vi "Enqueue.vi"(4 "Frist Call (F)":bool, 5 "QueueNames In":string[](array[string]), 6 "EnqueueType (QMH)":T2, 7 "EnqueueType (Enqueue)":T1=enum."Enqueue", 8 "error in (no error)":errorcluster, 9 "Message Data":variant, 10 "Message":string, 11 "Queue Array Reference In":refnum<queue>[](array[refnum])) -> (0 "error out":errorcluster, 2 "Queue Array Reference Out":refnum<queue>[](array[refnum]), 3 "MessageQueue":refnum<queue>)   [LabVIEW 2018, in "ScopePlugins.lvlib"]
uses:
  ScopePlugins.lvlib
  clMessage.ctl
  TypeDefs/QueueNames.ctl
  EnqueueTypes.ctl
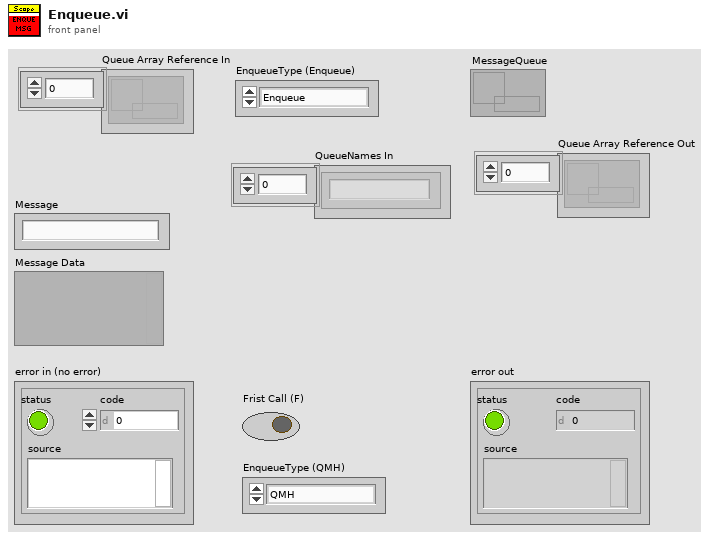
[diagram p1: front panel]
types:
  T1 = typedef "ScopePlugins.lvlib/EnqueueTypes.ctl" = enum16{"LossyEnqueue", "EnqueueAtFront", "Enqueue"}
  T2 = typedef "ScopePlugins.lvlib/QueueNames.ctl" = enum16{"QMH", "Class ", "MA"}
  T3 = typedef "ScopePlugins.lvlib/clMessage.ctl" = cluster{"Message":string, "Message Data":variant}
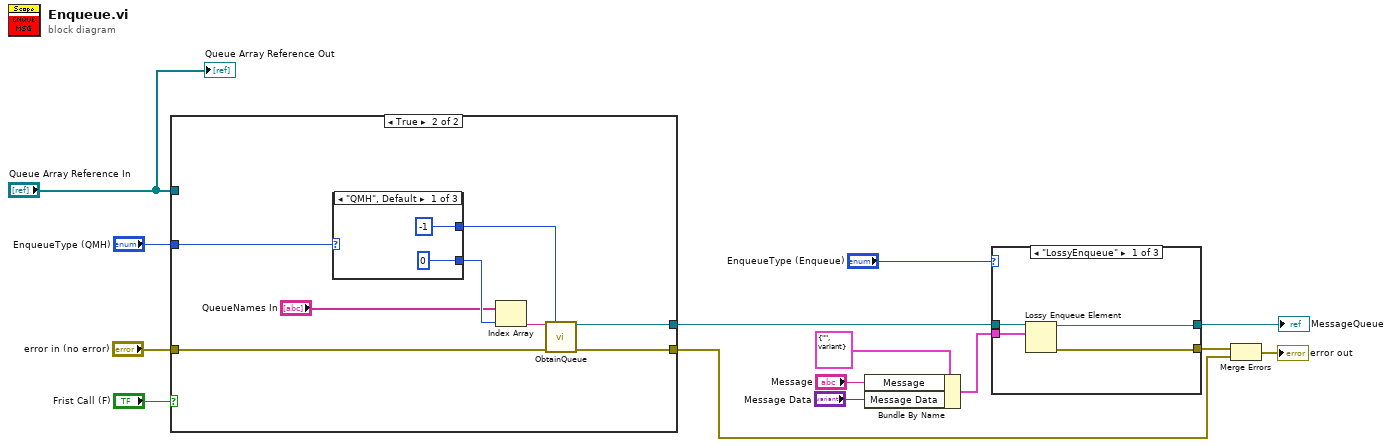
[diagram p0: block diagram]
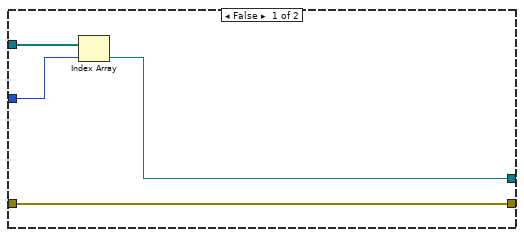
[diagram p2: hidden frame]
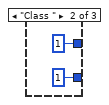
[diagram p3: hidden frame]
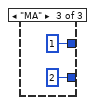
[diagram p4: hidden frame]
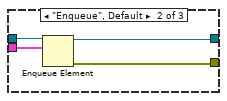
[diagram p5: hidden frame]
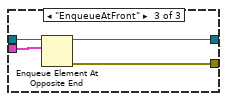
[diagram p6: hidden frame]
diagram:
  n1 = case shown="True" "Frist Call (F)" {
    tunnel: [w17 w26] -> w7
    tunnel: [w16 w25] -> w6
    tunnel: "EnqueueType (QMH)" -> [w18 w20]
    tunnel: "error in (no error)" -> [w16 w19]
    tunnel: "Queue Array Reference In" -> [w15 _]
    frame False {
      n2 = Index Array(array=w15, index=w18) -> (element=w17:refnum<queue>)
    }
    frame True {
      n3 = case shown="\"QMH\", Default" w20 {
        tunnel: [-1 ("max queue size (-1, unlimited)") 1 ("max queue size (-1, unlimited)") 1 ("max queue size (-1, unlimited)")] -> w24
        tunnel: [0 ("Queue Name Index (0) 2") 1 ("Queue Name Index (0) 2") 2 ("Queue Name Index (0) 2")] -> w23
        frame "QMH", Default {
        }
        frame "Class " {
        }
        frame "MA" {
        }
      }
      n4 = Index Array(array="QueueNames In", index=w23) -> (element=w22:string)
      n5 = call "ObtainQueue.vi"("Queue Name"=w22, "max queue size (-1, unlimited)"=w24, "error in (no error)"=w19) -> ("MessageQueue"=w26:refnum<queue>, "error out"=w25:errorcluster)  [unwired: 11 in]
    }
  }
  n6 = Bundle By Name(cluster=T3 {"Message"="", "Message Data"=variant} ("clMessage"), "Message"="Message", "Message Data"="Message Data") -> (w13:T3)
  n7 = case shown="\"LossyEnqueue\"" "EnqueueType (Enqueue)" {
    tunnel: w13 -> [w35 w39 w44]
    tunnel: w7 -> [w36 w40 w43]
    tunnel: [w33 w37 w42] -> w10
    tunnel: [w34 w38 w41] -> w8
    frame "LossyEnqueue" {
      n8 = Lossy Enqueue Element(queue=w36, element=w35) -> (queue out=w33:refnum<queue>, error out=w34:errorcluster)  [unwired: 1 in, 2 out]
    }
    frame "Enqueue", Default {
      n9 = Enqueue Element(queue=w40, element=w39) -> (queue out=w37:refnum<queue>, error out=w38:errorcluster)  [unwired: 2 in, 1 out]
    }
    frame "EnqueueAtFront" {
      n10 = Enqueue Element At Opposite End(queue=w43, element=w44) -> (queue out=w42:refnum<queue>, error out=w41:errorcluster)  [unwired: 2 in, 1 out]
    }
  }
  "MessageQueue" <- w10
  n11 = Merge Errors(w8, w6) -> (→"error out":errorcluster)
  "Queue Array Reference Out" <- "Queue Array Reference In"
